vi "Write Direct Message Msg.vi"(10 "Chat Window UI Controller.lvlib:Direct Message Msg.lvclass":refnum<class "Direct Message Msg.lvclass">, 11 "Chat Window UI Controller in":refnum<class "Chat Window UI Controller.lvclass">) -> (3 "Chat Window UI Controller out":refnum<class "Chat Window UI Controller.lvclass">)   [LabVIEW 2018, in "Chat Window UI Controller.lvlib" / "Chat Window UI Controller.lvclass"]
uses:
  Chat Window UI Controller.lvclass
  Chat Window UI Controller Messages/Direct Message Msg/Direct Message Msg.lvclass
  Chat Window UI Controller.lvclass/Chat Window UI Controller.ctl
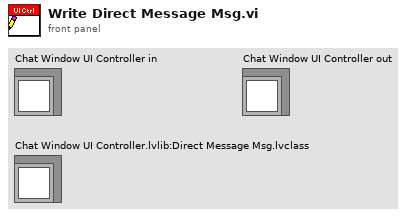
[diagram p1: front panel]
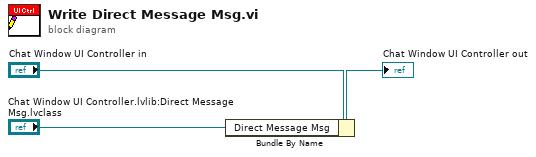
[diagram p0: block diagram]
diagram:
  n1 = Bundle By Name(cluster="Chat Window UI Controller in", "Direct Message Msg"="Chat Window UI Controller.lvlib:Direct Message Msg.lvclass") -> (→"Chat Window UI Controller out":refnum<class "Chat Window UI Controller.lvclass">)
